vi "1-x_to_2-x.vi"(1 "Кол-во копий":i32=5, 2 "Размер окна":i32=4, 3 "Входной одномерный массив":dbl[](array[numeric])) -> (0 "Двухмерный массив":dbl[][](array[numeric]))   [LabVIEW 2017]
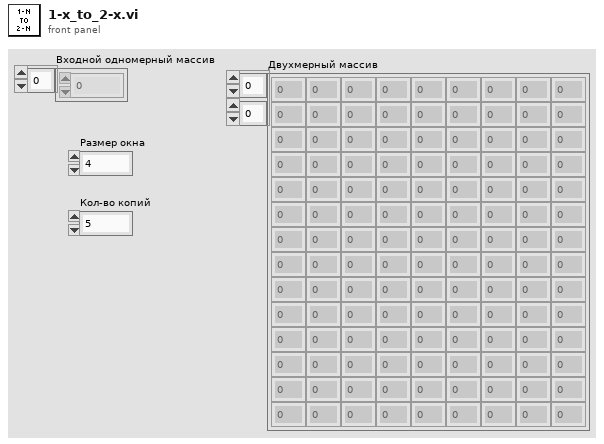
[diagram p1: front panel]
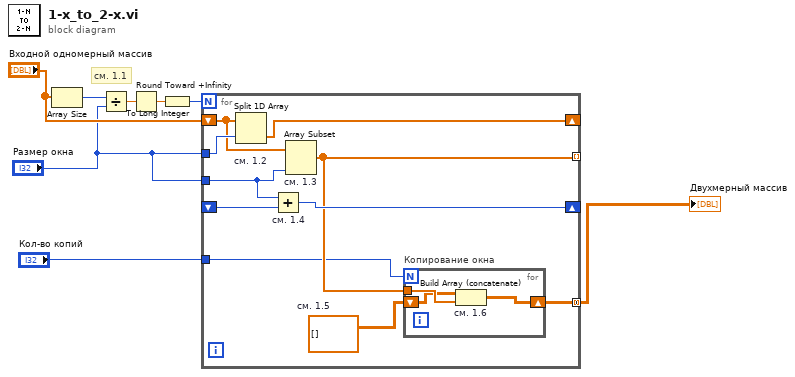
[diagram p0: block diagram]
diagram:
  # "см. 1.1"
  n1 = Array Size(array="Входной одномерный массив") -> (size(s)=w5:i32)
  n2 = Divide(x=w5, y="Размер окна") -> (x/y=w6:dbl)
  n3 = Round Toward +Infinity(x=w6) -> (ceil(x): smallest int >= x=w7:dbl)
  n4 = To Long Integer(number=w7) -> (32bit integer=w8:i32)
  n5 = for {
    N: w8 -> [_]
    shift-right: [w18] -> _
    shift-left: "Входной одномерный массив" -> [w16]
    tunnel: "Размер окна" -> [w17]
    shift-right: [w14] -> _
    shift-left: _ -> [w13]
    tunnel: "Размер окна" -> [w15]
    tunnel: [w12] -> _ mode=indexing
    tunnel: [w11] -> w4 mode=concatenating
    tunnel: "Кол-во копий" -> [w9]
    w10 = dbl[][] []  # см. 1.5
    n6 = Split 1D Array "см. 1.2"(array=w16, index=w17) -> (second subarray=w18:dbl[])  [unwired: 1 out]
    n7 = Add "см. 1.4"(x=w15, y=w13) -> (x+y=w14:i32)
    n8 = Array Subset "см. 1.3"(array=w16, length=w15) -> (w12:dbl[])  [unwired: 1 in]
    n9 = for "Копирование окна" {
      N: w9 -> [_]
      tunnel: w12 -> [w20]
      shift-right: [w21] -> w11
      shift-left: w10 -> [w19]
      n10 = Build Array (concatenate) "см. 1.6"(w19, w20) -> (w21:dbl[][])
    }
  }
  "Двухмерный массив" <- w4
